vi "Collect information from UI to run measurement.vi"(8 "error in (no error)":errorcluster, 11 "Measurement UI in":refnum<class "Measurement UI.lvclass">) -> (0 "error out":errorcluster, 1 "Show UI?":bool, 2 "Device Names":string[](array[string]), 3 "Measurement UI out":refnum<class "Measurement UI.lvclass">, 4 "String":string, 5 "Measurement Name":string, 6 "Run continuously?":bool)   [LabVIEW 2016, in "Measurement UI.lvlib" / "Measurement UI.lvclass"]
uses:
  Measurement UI.lvclass
  Measurement UI.lvclass/Measurement UI.ctl
  Accessors/Read Measurement.vi
  Accessors/Read Power Supply.vi
  Accessors/Read Digitizer.vi
  Accessors/Read Function Generator.vi
  Read Multimeter.vi
  Accessors/Read Show FP_.vi
  Read Run Indefinitely.vi
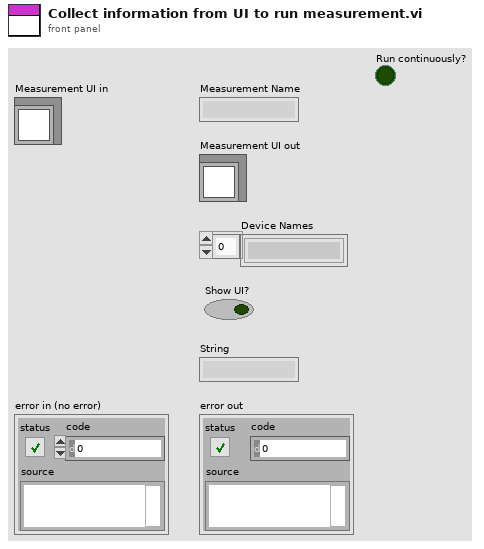
[diagram p1: front panel]
types:
  T1 = enum8{"Enabled", "Disabled", "Disabled and Grayed Out"}
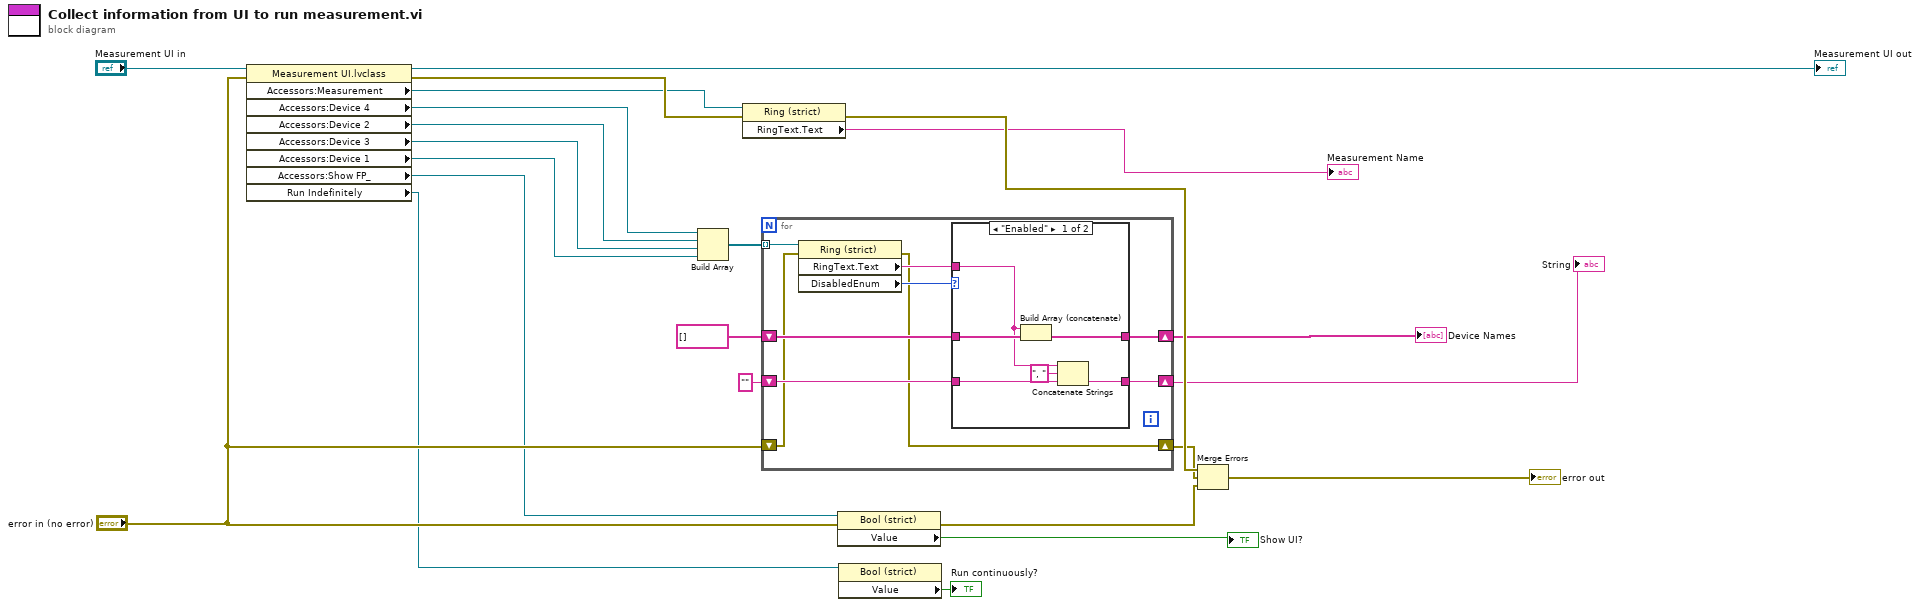
[diagram p0: block diagram]
diagram:
  n1 = property class="Measurement UI.lvclass"(reference="Measurement UI in", error in="error in (no error)") -> (reference out=→"Measurement UI out":refnum<class "Measurement UI.lvclass">, error out=w18:errorcluster, "Accessors:Measurement"=w17:refnum<vi>, "Accessors:Device 4"=w16:refnum<vi>, "Accessors:Device 2"=w15:refnum<vi>, "Accessors:Device 3"=w14:refnum<vi>, "Accessors:Device 1"=w13:refnum<vi>, "Accessors:Show FP_"=w12:refnum<vi>, "Run Indefinitely"=w2:refnum<vi>)
  n2 = Build Array(w16, w15, w14, w13) -> (w5:refnum<vi>[])
  n3 = property class="Ring (strict)"(reference=w17, error in=w18) -> (error out=w22:errorcluster, "RingText.Text"=→"Measurement Name":string)  [unwired: 1 out]
  n4 = for {
    shift-right: [w29] -> w4
    shift-left: string[] [] ("Device Names") -> [w28]
    tunnel: w5 -> [w32] mode=indexing
    shift-right: [w27] -> w9
    shift-left: "" -> [w26]
    shift-right: [w25] -> w20
    shift-left: "error in (no error)" -> [w24]
    n5 = property class="Ring (strict)"(reference=w32, error in=w24) -> (error out=w25:errorcluster, "RingText.Text"=w30:string, "DisabledEnum"=w31:T1)  [unwired: 1 out]
    n6 = case shown="\"Enabled\"" w31 {
      tunnel: w30 -> [w34 _]
      tunnel: [w38 w40] -> w29
      tunnel: w28 -> [w37 w40]
      tunnel: [w36 w39] -> w27
      tunnel: w26 -> [w35 w39]
      frame "Enabled" {
        n7 = Build Array (concatenate)(w34, w37) -> (w38:string[])
        n8 = Concatenate Strings(w34, ", " ("string"), w35) -> (w36:string)
      }
      frame "Disabled", Default {
      }
    }
  }
  "String" <- w9
  "Device Names" <- w4
  n9 = property class="Bool (strict)"(reference=w12, error in="error in (no error)") -> (error out=w21:errorcluster, "Value"=→"Show UI?":bool)  [unwired: 1 out]
  n10 = property class="Bool (strict)"(reference=w2) -> ("Value"=→"Run continuously?":bool)  [unwired: 1 in, 2 out]
  n11 = Merge Errors(w22, w20, w21) -> (→"error out":errorcluster)
